vi "global stop1.vi"() -> ()   [LabVIEW 2020]
panel:
  in  "global stop":bool
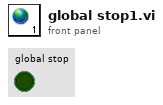
[diagram p1: front panel]
diagram:
